vi "PB_reset.vi"(3 "Path to spinapi.dll":path=path "C:/SpinCore/SpinAPI/dll/spinapi.dll") -> ()   [LabVIEW 2012]
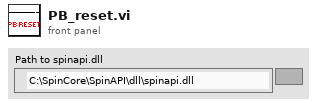
[diagram p1: front panel]
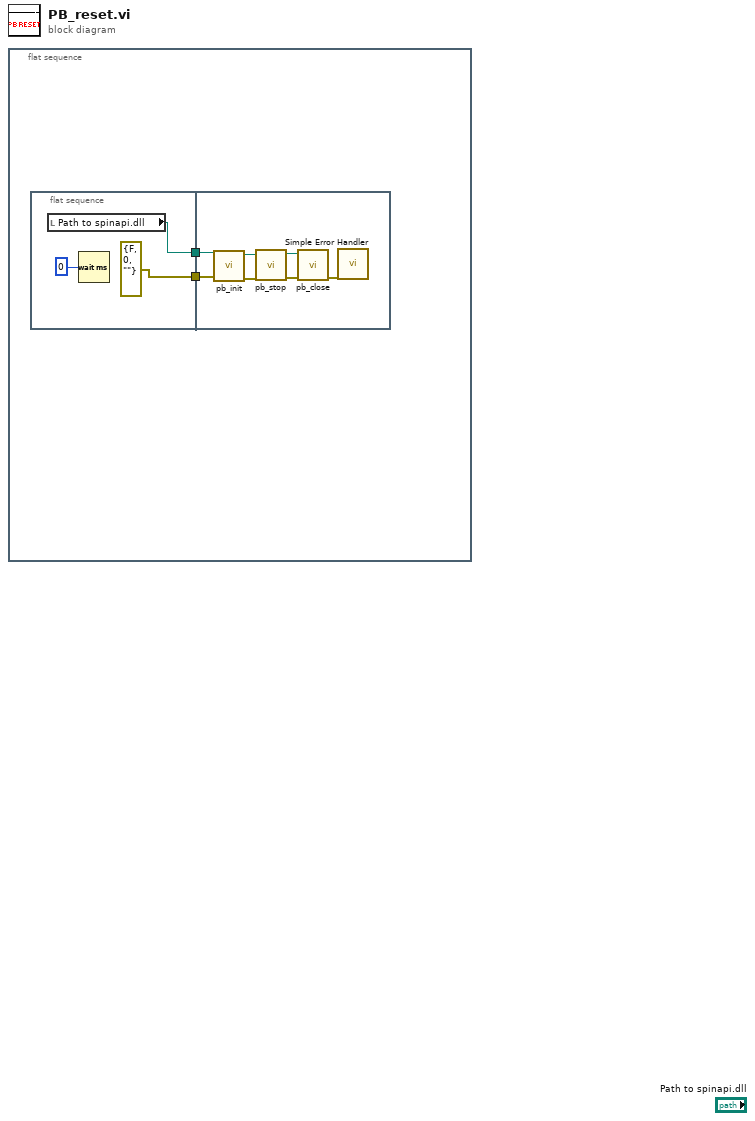
[diagram p0: block diagram]
diagram:
  n1 = flat-sequence {
    frame #0 {
      n2 = flat-sequence {
        tunnel: [errorcluster {"status"=FALSE, "code"=0, "source"=""} ("error in (no error)")] -> w2
        tunnel: [w3] -> w1
        tunnel: w2 -> [w7]
        tunnel: w1 -> [w8]
        frame #0 {
          n3 = local read "Path to spinapi.dll"() -> (w3:path)
          n4 = Wait (ms)(milliseconds to wait=u32 0) -> ()  [unwired: 1 out]
        }
        frame #1 {
          n5 = call "pb_init.vi"("error in (no error)"=w7, "path in"=w8) -> ("error out"=w11:errorcluster, "path out"=w12:path)  [unwired: 8 in]
          n6 = call "pb_stop.vi"("error in (no error)"=w11, "path in"=w12) -> ("error out"=w9:errorcluster, "path out"=w10:path)  [unwired: 8 in]
          n7 = call "pb_close.vi"("error in (no error)"=w9, "path in"=w10) -> ("error out"=w6:errorcluster)  [unwired: 9 out]
          n8 = call <vilib>:"Simple Error Handler.vi"("error in (no error)"=w6) -> ()  [unwired: 1 in, 8 out]
        }
      }
    }
  }
